vi "Pre Initialzie.vi"(6 "publishing interval (10 ms)":dbl=10.0 format="%#_13g", 8 "error in (no error)":errorcluster, 10 "SUbscription Node IDs":string, 11 "Model in":refnum<class "Model.lvclass">) -> (0 "error out":errorcluster, 3 "Model out":refnum<class "Model.lvclass">, 5 "OPCUA Even":T2, 7 "Evens":T1)   [LabVIEW 2021, in "Model.lvlib" / "Model.lvclass"]
uses:
  Model.lvclass
  <userlib>/John_Lib/OPCUA/OPCUA Even.ctl
  <vilib>/OPCUA/controls/Subscription Data Change.ctl
  <vilib>/OPCUA/controls/NodeId.ctl
  <vilib>/OPCUA/controls/Data Type.ctl
  <vilib>/OPCUA/controls/OPC UA StatusCode.ctl
  <vilib>/OPCUA/controls/Subscription ID.ctl
  <userlib>/John_Lib/OPCUA/ReSubscription Even.ctl
  Evens.ctl
  DVR.ctl
  <userlib>/John_Lib/Network_Streams_Connection/NetworkConnection.lvclass
  AMC Q.ctl
  <userlib>/John_Lib/AMC_FW/AMC_SelfCustom/Queue.ctl
  <userlib>/John_Lib/AMC_FW/Message Queue.ctl
  <userlib>/John_Lib/AMC_FW/Message.ctl
  <userlib>/John_Lib/AMC_FW/Tools/Keyed Array/KeyedArray.ctl
  Model.lvclass/Model.ctl
  <userlib>/John_Lib/OPCUA/OPCUA.lvclass
  <userlib>/John_Lib/AMC_FW/AMC_FW.lvlib
  <userlib>/John_Lib/AMC_FW/Tools/Keyed Array/Tools_KeyedArray.lvlib
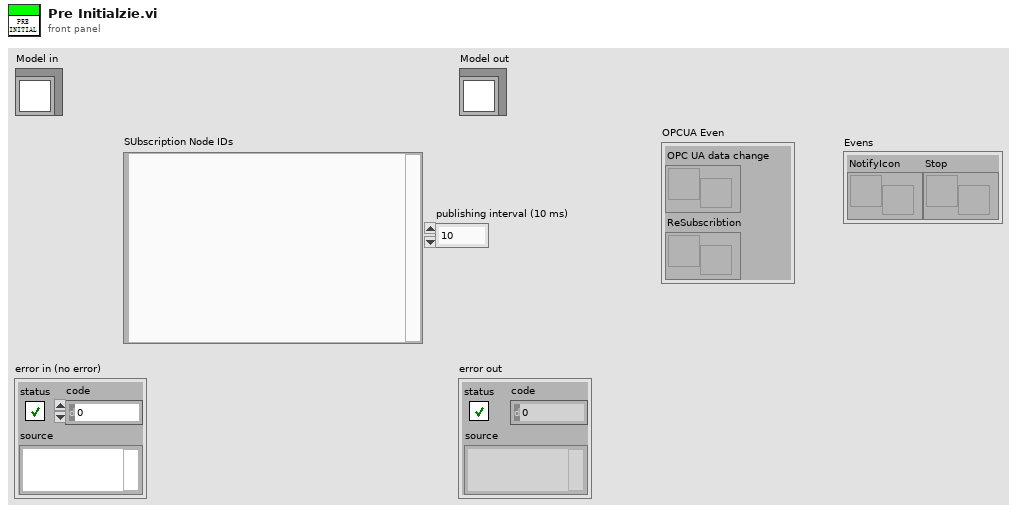
[diagram p1: front panel]
types:
  T1 = typedef "Model.lvlib/Model.lvclass/Evens.ctl" = cluster{"NotifyIcon":refnum<user-event>, "Stop":refnum<user-event>}
  T2 = typedef "OPCUA.lvlib/OPCUA.lvclass/OPCUA Even.ctl" = cluster{"OPC UA data change":refnum<user-event>, "ReSubscribtion":refnum<user-event>}
  T3 = typedef "Model.lvlib/Model.lvclass/DVR.ctl" = cluster{"JKI_Network_Streams":refnum<class "NetworkConnection.lvclass">, "AMC Q":T4}
  T4 = typedef "Model.lvlib/Model.lvclass/AMC Q.ctl" = cluster{"Main":T5, "OPCUA":T5, "NetworkSteam":T5}
  T5 = typedef "AMC_FW.lvlib/Queue.ctl" = cluster{"Q":T6, "Name":string}
  T6 = typedef "AMC_FW.lvlib/Message Queue.ctl" = refnum<queue>
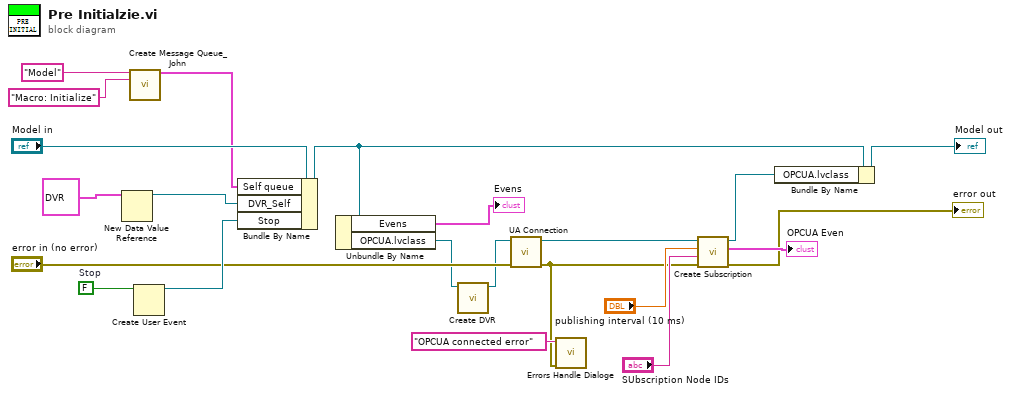
[diagram p0: block diagram]
diagram:
  w21 = FALSE  # Stop
  n1 = New Data Value Reference(data value=T3 {"JKI_Network_Streams"=refnum, "AMC Q"={"Main"={"Q"=refnum, "Name"=""}, "OPCUA"={"Q"=refnum, "Name"=""}, "NetworkSteam"={"Q"=refnum, "Name"=""}}} ("DVR")) -> (data value reference=w1:refnum<data-value>)  [unwired: 1 in, 1 out]
  n2 = call <userlib>:"Create Message Queue_John.vi"("message queue name"="Model", "initial message names"="Macro: Initialize") -> ("message queue out"=w5:T5)  [unwired: 12 in, 1 out]
  n3 = Create User Event(user event datatype=w21) -> (user event=w20:refnum<user-event>)  [unwired: 1 in, 1 out]
  n4 = Bundle By Name(cluster="Model in", "Self queue"=w5, "DVR_Self"=w1, "Stop"=w20) -> (w19:refnum<class "Model.lvclass">)
  n5 = Unbundle By Name(w19) -> ("Evens"=→"Evens":T1, "OPCUA.lvclass"=w4:refnum<class "OPCUA.lvclass">)
  n6 = call <userlib>:"Create DVR.vi"("OPCUA in"=w4) -> ("OPCUA out"=w3:refnum<class "OPCUA.lvclass">)  [unwired: 9 in, 1 out]
  n7 = call <userlib>:"UA Connection.vi"("error in (no error)"="error in (no error)", "OPCUA in"=w3) -> ("error out"=w10:errorcluster, "OPCUA out"=w17:refnum<class "OPCUA.lvclass">)  [unwired: 8 in]
  n8 = call <userlib>:"Errors Handle Dialoge.vi"("error in (no error)"=w10, "Message"="OPCUA connected error") -> ()  [unwired: 8 in, 2 out]
  n9 = call <userlib>:"Create Subscription.vi"("error in (no error)"=w10, "Node IDs"="SUbscription Node IDs", "publishing interval (10 ms)"="publishing interval (10 ms)", "OPCUA in"=w17) -> ("error out"=→"error out":errorcluster, "Even"=→"OPCUA Even":T2, "OPCUA out"=w13:refnum<class "OPCUA.lvclass">)  [unwired: 5 in]
  n10 = Bundle By Name(cluster=w19, "OPCUA.lvclass"=w13) -> (→"Model out":refnum<class "Model.lvclass">)
